vi "ASSIGNMENT OF SEVEN SEGMENT DISPLAY.vi"() -> ()   [LabVIEW 2018]
panel:
  in  "Dial":u8(knob) scale=0.0..9.0
  out "D":bool
  out "E":bool
  out "C":bool
  out "G":bool
  out "F":bool
  out "B":bool
  out "A":bool
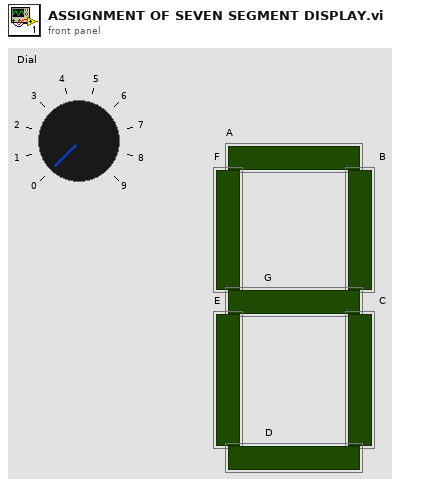
[diagram p1: front panel]
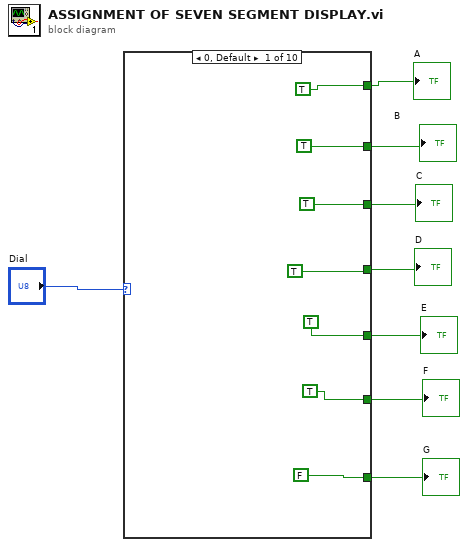
[diagram p0: block diagram]
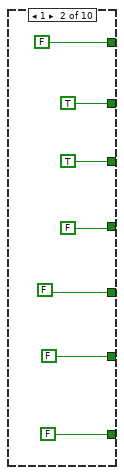
[diagram p2: hidden frame]
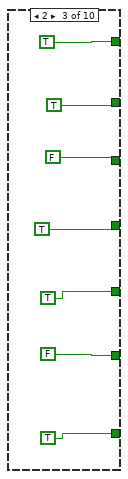
[diagram p3: hidden frame]
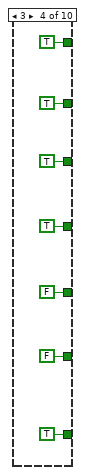
[diagram p4: hidden frame]
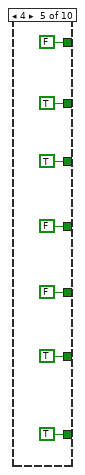
[diagram p5: hidden frame]
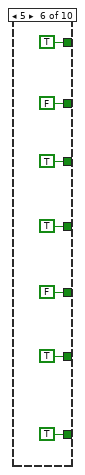
[diagram p6: hidden frame]
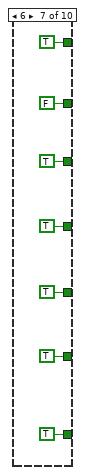
[diagram p7: hidden frame]
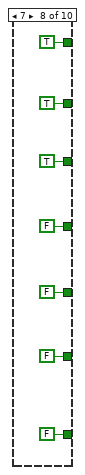
[diagram p8: hidden frame]
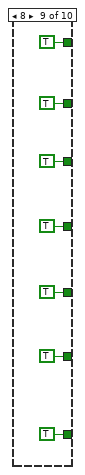
[diagram p9: hidden frame]
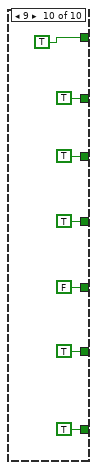
[diagram p10: hidden frame]
diagram:
  n1 = case shown="0, Default" "Dial" {
    tunnel: [TRUE FALSE TRUE TRUE FALSE TRUE TRUE TRUE TRUE TRUE] -> w4
    tunnel: [TRUE TRUE TRUE TRUE TRUE FALSE FALSE TRUE TRUE TRUE] -> w3
    tunnel: [TRUE TRUE FALSE TRUE TRUE TRUE TRUE TRUE TRUE TRUE] -> w2
    tunnel: [TRUE FALSE TRUE FALSE FALSE FALSE TRUE FALSE TRUE FALSE] -> w1
    tunnel: [TRUE FALSE FALSE FALSE TRUE TRUE TRUE FALSE TRUE TRUE] -> w8
    tunnel: [FALSE FALSE TRUE TRUE TRUE TRUE TRUE FALSE TRUE TRUE] -> w7
    tunnel: [TRUE FALSE TRUE TRUE FALSE TRUE TRUE FALSE TRUE TRUE] -> w6
    frame 0, Default {
    }
    frame 1 {
    }
    frame 2 {
    }
    frame 3 {
    }
    frame 4 {
    }
    frame 5 {
    }
    frame 6 {
    }
    frame 7 {
    }
    frame 8 {
    }
    frame 9 {
    }
  }
  "B" <- w3
  "C" <- w2
  "A" <- w4
  "D" <- w6
  "E" <- w1
  "F" <- w8
  "G" <- w7
